vi "GetCurrentStatus.vi"() -> ()   [LabVIEW 2018]
panel:
  out "error out":errorcluster caption="错误输出"
  in  "error in (no error)":errorcluster caption="错误输入（无错误）"
  in  "VISA资源名称输出":refnum<visa-resource-name>
  in  "VISA资源名称输入":refnum<visa-resource-name>
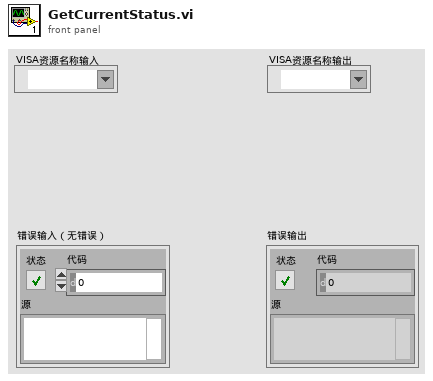
[diagram p1: front panel]
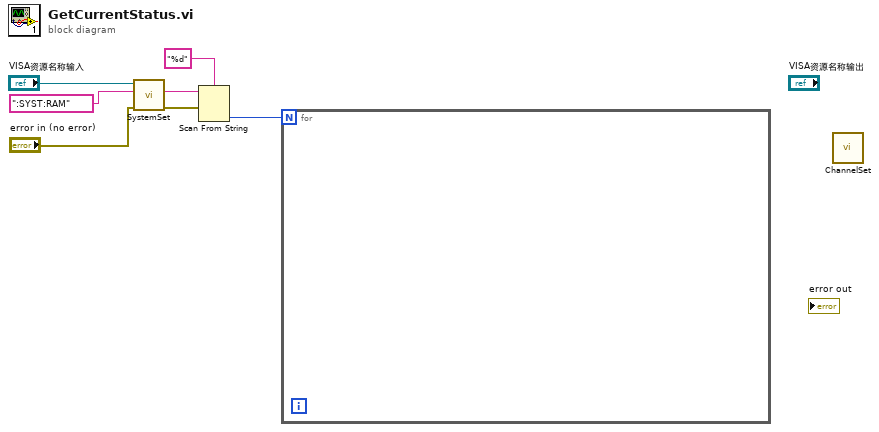
[diagram p0: block diagram]
diagram:
  n1 = call "SystemSet.vi"("error in (no error)"="error in (no error)", "SYSTEM命令子系统"=":SYST:RAM", "VISA资源名称"="VISA资源名称输入") -> ("error out"=w3:errorcluster, "查询返回"=w4:string)  [unwired: 5 in, 2 out]
  n2 = Scan From String(format string="%d" ("格式字符串"), input string=w4, error in=w3) -> (output 1=w1:i32)  [unwired: 2 in, 3 out]
  n3 = for {
    N: w1 -> [_]
  }
  n4 = call "ChannelSet.vi"() -> ()  [unwired: 8 in, 4 out]
